vi "HV Error Statuses.vi"(11 "transposed array":string[][](array[string])) -> (3 "Status Errors":string[](array[string]))   [LabVIEW 2018, in "HV QMH.lvlib"]
uses:
  HV QMH.lvlib
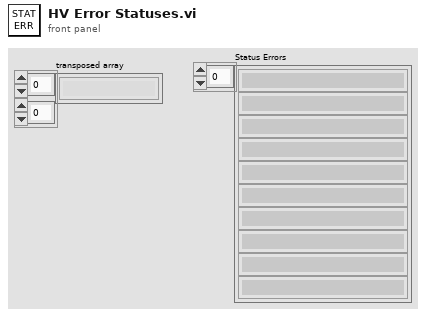
[diagram p1: front panel]
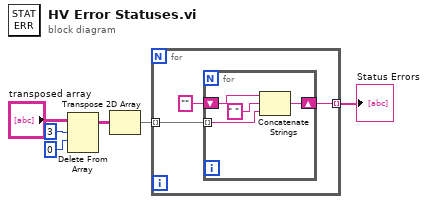
[diagram p0: block diagram]
diagram:
  n1 = Delete From Array(array="transposed array", length=3, index (row)=0 ("index")) -> (array with subset deleted=w5:string[][])  [unwired: 1 in, 1 out]
  n2 = Transpose 2D Array(2D array=w5) -> (transposed array=w6:string[][])
  n3 = for {
    tunnel: w6 -> [w9] mode=indexing
    tunnel: [w7] -> w1 mode=indexing
    n4 = for {
      tunnel: w9 -> [w11] mode=indexing
      shift-right: [w13] -> w7
      shift-left: "" -> [w12]
      n5 = Concatenate Strings(w12, " " ("string"), w11) -> (w13:string)
    }
  }
  "Status Errors" <- w1
